vi "Insert Menu.vi"(7 "Run Mode?":bool, 8 "error in (no error)":errorcluster, 9 "Active Plot ID":i32, 10 "Plot Names":string[](array[string]), 11 "MenuRef":refnum<k9>) -> (0 "error out":errorcluster, 3 "Dup MenuRef":refnum<k9>)   [LabVIEW 2020, in "3D Plot.lvclass"]
uses:
  3D Plot.lvclass
panel:
  in  "Root Item Runmode":string[](array[string])=["Render Window", "3D Plot Properties"]
  in  "Snap Item Names":string[](array[string])=["Export to File...", "Export to Printer"]
  in  "Root Item Names":string[](array[string])=["Active Plot", "Export Image", "Render Window", "3D Plot Properties", "", "Properties"]
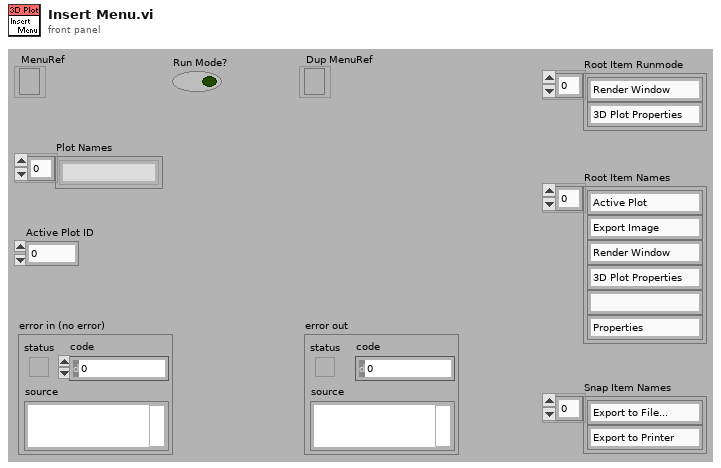
[diagram p1: front panel]
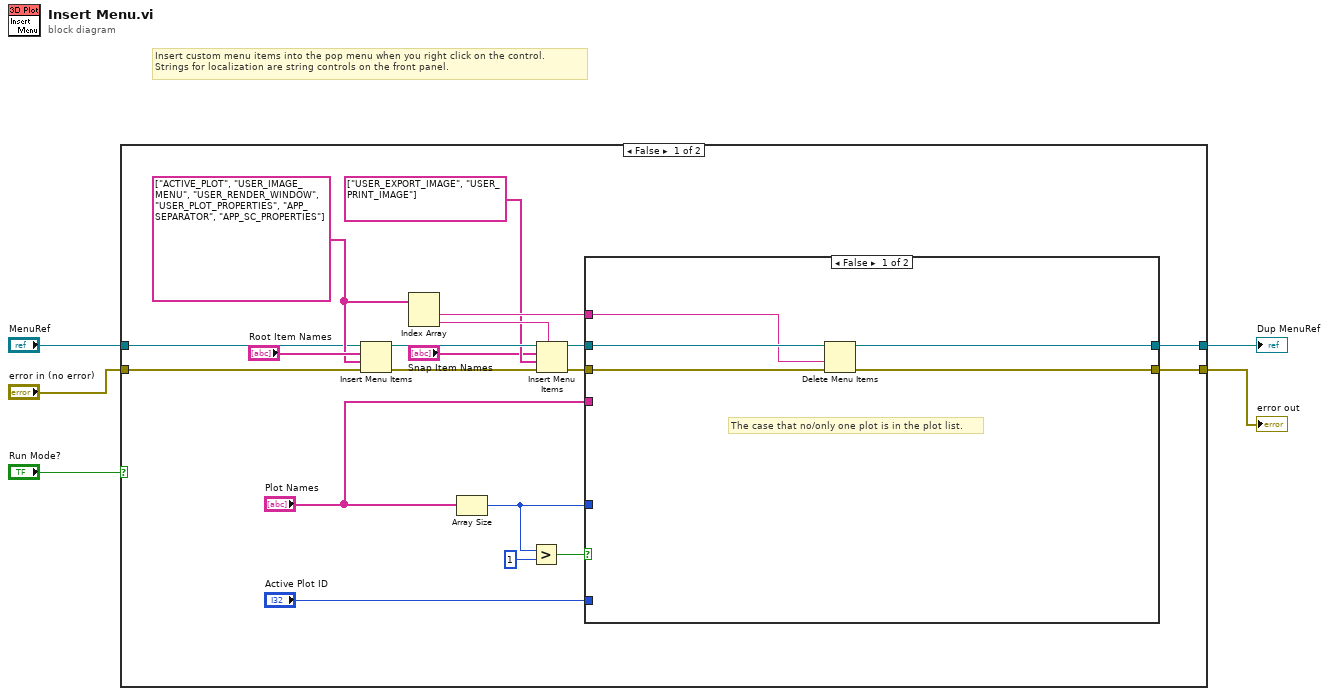
[diagram p0: block diagram]
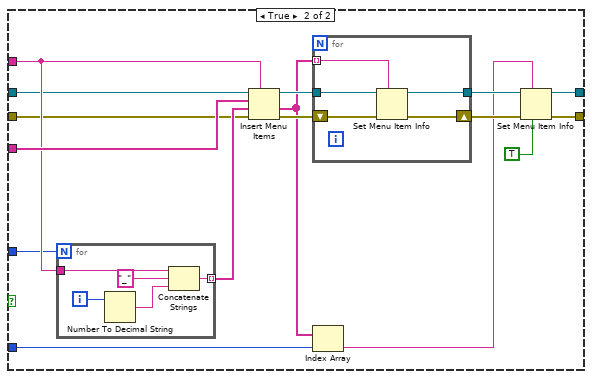
[diagram p2: hidden frame]
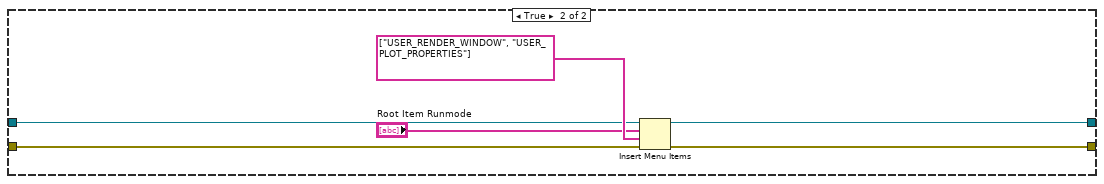
[diagram p3: hidden frame]
diagram:
  # "Insert custom menu items into the pop menu when you right click on the control.\nStrings for localization are string controls on the front panel."
  n1 = case shown="False" "Run Mode?" {
    tunnel: [w21 w59] -> w5
    tunnel: [w19 w58] -> w4
    tunnel: "MenuRef" -> [w11 w60]
    tunnel: "error in (no error)" -> [w10 w57]
    frame False {
      w23 = string[] ["ACTIVE_PLOT", "USER_IMAGE_MENU", "USER_RENDER_WINDOW", "USER_PLOT_PROPERTIES", "APP_SEPARATOR", "APP_SC_PROPERTIES"] ("item names")
      n2 = Insert Menu Items(6:w10, 7:w23, 8:"Root Item Names", 9:w11) -> (0:w15:errorcluster, 3:w18:refnum<k9>)  [unwired: 3 out]
      n3 = Index Array(array=w23) -> (element #1=w22:string, element #2=w16:string)  [unwired: 2 in]
      n4 = Array Size(array="Plot Names") -> (size(s)=w6:i32)
      n5 = Greater?(x=w6, y=1) -> (0:w7:bool)
      n6 = Insert Menu Items(5:w16, 6:w15, 7:string[] ["USER_EXPORT_IMAGE", "USER_PRINT_IMAGE"] ("item names"), 8:"Snap Item Names", 9:w18) -> (0:w14:errorcluster, 3:w17:refnum<k9>)  [unwired: 1 in, 1 out]
      n7 = case shown="False" w7 {
        tunnel: "Plot Names" -> [_ w45]
        tunnel: w22 -> [w25 w44]
        tunnel: [w28 w41] -> w21
        tunnel: "Active Plot ID" -> [_ w36]
        tunnel: [w26 w34] -> w19
        tunnel: w17 -> [w29 w32]
        tunnel: w14 -> [w27 w31]
        tunnel: w6 -> [_ w30]
        frame False {
          # "The case that no/only one plot is in the plot list."
          n8 = Delete Menu Items(6:w27, 7:w25, 9:w29) -> (0:w26:errorcluster, 3:w28:refnum<k9>)  [unwired: 1 in]
        }
        frame True {
          n9 = for {
            N: w30 -> [_]
            tunnel: w44 -> [w55]
            tunnel: [w51] -> w43 mode=indexing
            i -> [w52]
            n10 = Number To Decimal String(number=w52) -> (decimal integer string=w53:string)  [unwired: 1 out]
            n11 = Concatenate Strings(w55, "_" ("string"), w53) -> (w51:string)
          }
          n12 = Insert Menu Items(5:w44, 6:w31, 7:w43, 8:w45, 9:w32) -> (0:w39:errorcluster, 1:w37:string[], 3:w42:refnum<k9>)  [unwired: 1 in]
          n13 = for {
            tunnel: w42 -> [w50]
            tunnel: [w49] -> w40
            tunnel: w37 -> [w48] mode=indexing
            shift-right: [w46] -> w38
            shift-left: w39 -> [w47]
            n14 = Set Menu Item Info(7:w48, 8:w47, 11:w50) -> (0:w46:errorcluster, 3:w49:refnum<k9>)  [unwired: 4 out]
          }
          n15 = Index Array(array=w37, index=w36) -> (element=w35:string)
          n16 = Set Menu Item Info(6:TRUE ("checked"), 7:w35, 8:w38, 11:w40) -> (0:w34:errorcluster, 3:w41:refnum<k9>)  [unwired: 3 out]
        }
      }
    }
    frame True {
      n17 = Insert Menu Items(6:w57, 7:string[] ["USER_RENDER_WINDOW", "USER_PLOT_PROPERTIES"] ("item names"), 8:"Root Item Runmode", 9:w60) -> (0:w58:errorcluster, 3:w59:refnum<k9>)  [unwired: 3 out]
    }
  }
  "error out" <- w4
  "Dup MenuRef" <- w5
